vi "Switch.vi"(8 "error in (no error)":errorcluster, 10 "Parameters":string, 11 "reference in":refnum<class "Test_Flux_Capacitor.lvclass">) -> (0 "error out":errorcluster, 2 "Result":bool, 3 "reference out":refnum<class "Test_Flux_Capacitor.lvclass">)   [LabVIEW 2022 SP3, in "Test_Flux_Capacitor.lvlib" / "Test_Flux_Capacitor.lvclass"]
uses:
  Test_Flux_Capacitor.lvclass
  ParameterTypes/PowerDUT.ctl
  <vilib>/Utility/error.llb/Trim Whitespace One-Sided.vi
  Components/SwitchBase.lvlibp/SwitchBase.lvclass
  <vilib>/JDP Science/JSONtext/JSONtext.lvlib
panel:
  in  "Parameter_Type":T1
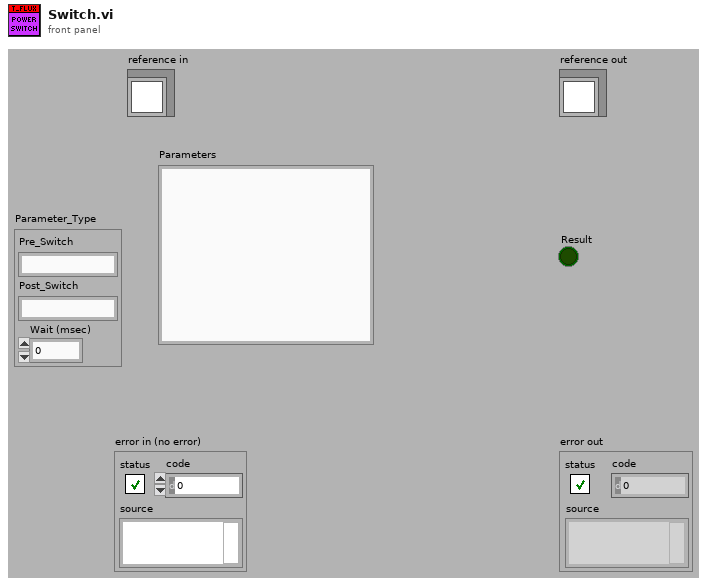
[diagram p1: front panel]
types:
  T1 = typedef "Test_Flux_Capacitor.lvlib/Test_Flux_Capacitor.lvclass/PowerDUT.ctl" = cluster{"Pre_Switch":string, "Post_Switch":string, "Wait (msec)":u32}
  T2 = typedef "Test_Flux_Capacitor.lvlib/Test_Flux_Capacitor.lvclass/ObjectAttributes.ctl" = cluster{"Config":T3, "DMM":refnum<class "DMM_Keysight_34980A.lvclass">, "LCR":refnum<class "LCR_BK891.lvclass">, "PSU":refnum<class "PSU_Base.lvclass">, "Switch_Manager":refnum<class "SwitchBase.lvclass">, "FRAM":string, "Flux_Capacitor":refnum<class "Flux_Capacitor.lvclass">, "Frequency_Counter":refnum<class "Frequency_Counter_Base.lvclass">, "JTAG":refnum<class "JTAG_Base.lvclass">}
  T3 = typedef "Test_Flux_Capacitor.lvlib/Test_Flux_Capacitor.lvclass/Config.ctl" = cluster{"default":string}
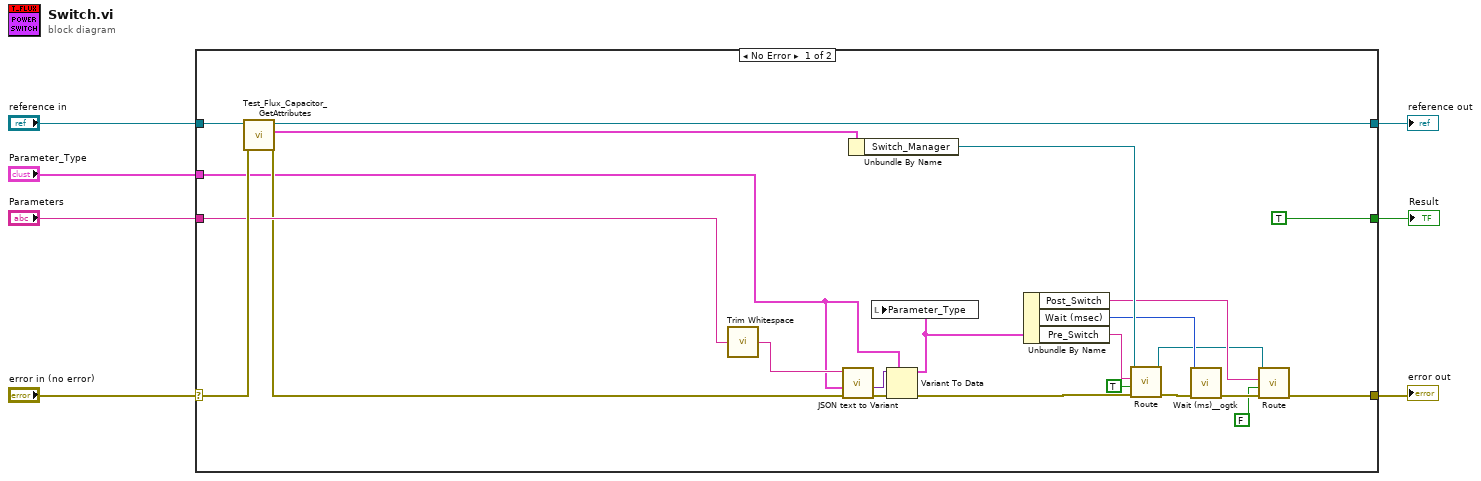
[diagram p0: block diagram]
diagram:
  n1 = case shown="No Error" "error in (no error)" {
    selector: "error in (no error)" -> [w30 w32]
    tunnel: [w11 w32] -> w6
    tunnel: [w28 w31] -> w4
    tunnel: "reference in" -> [w29 w31]
    tunnel: "Parameters" -> [w23 _]
    tunnel: "Parameter_Type" -> [w13 _]
    tunnel: [TRUE _] -> w1
    frame No Error {
      n2 = call "Test_Flux_Capacitor_GetAttributes.vi"("error in (no error)"=w30, "reference in"=w29) -> ("error out"=w17:errorcluster, "Data"=w27:T2, "reference out"=w28:refnum<class "Test_Flux_Capacitor.lvclass">)  [unwired: 6 in, 1 out]
      n3 = call <vilib>:"Trim Whitespace.vi"("string"=w23) -> ("trimmed string"=w24:string)  [unwired: 1 in]
      n4 = call <vilib>:"JSON text to Variant.vi"("error in (no error)"=w17, "Data Type"=w13, "JSON"=w24) -> ("error out"=w15:errorcluster, "Variant out"=w16:variant)  [unwired: 7 in]
      n5 = Unbundle By Name(w27) -> ("Switch_Manager"=w26:refnum<class "SwitchBase.lvclass">)
      n6 = Variant To Data(error in=w15, type=w13, Variant=w16) -> (data=w22:T1, error out=w19:errorcluster)
      n7 = local write "Parameter_Type"(w22) -> ()
      n8 = Unbundle By Name(w22) -> ("Post_Switch"=w10:string, "Wait (msec)"=w20:u32, "Pre_Switch"=w21:string)
      n9 = call-dynamic "Route.vi"("error in (no error)"=w19, "Connect"=TRUE, "channel 1"=w21, "reference in"=w26) -> ("error out"=w25:errorcluster, "reference in"=w9:refnum<class "SwitchBase.lvclass">)  [unwired: 6 in]
      n10 = call <userlib>:"Wait (ms)__ogtk.vi"("error in (no error)"=w25, "milliseconds to wait"=w20) -> ("error out"=w12:errorcluster)  [unwired: 8 in, 1 out]
      n11 = call-dynamic "Route.vi"("error in (no error)"=w12, "Connect"=FALSE, "channel 1"=w10, "reference in"=w9) -> ("error out"=w11:errorcluster)  [unwired: 6 in, 1 out]
    }
    frame Error {
    }
  }
  "Result" <- w1
  "error out" <- w6
  "reference out" <- w4
